vi "Abort All Top Level in App Instance.vi"() -> ()   [LabVIEW 2020]
panel:
  in  "Select":bool
  in  "Contexts":i32(listbox)
  out "error out":errorcluster
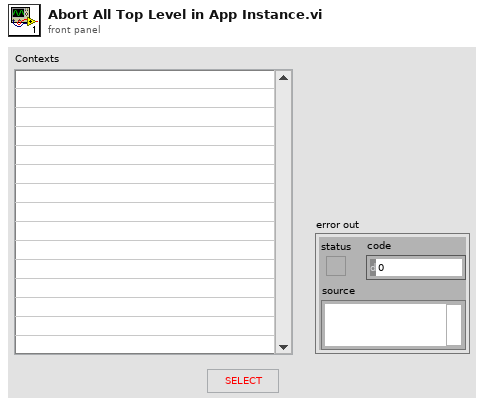
[diagram p1: front panel]
types:
  T1 = enum32{"Bad", "Idle", "Run top level", "Running"}
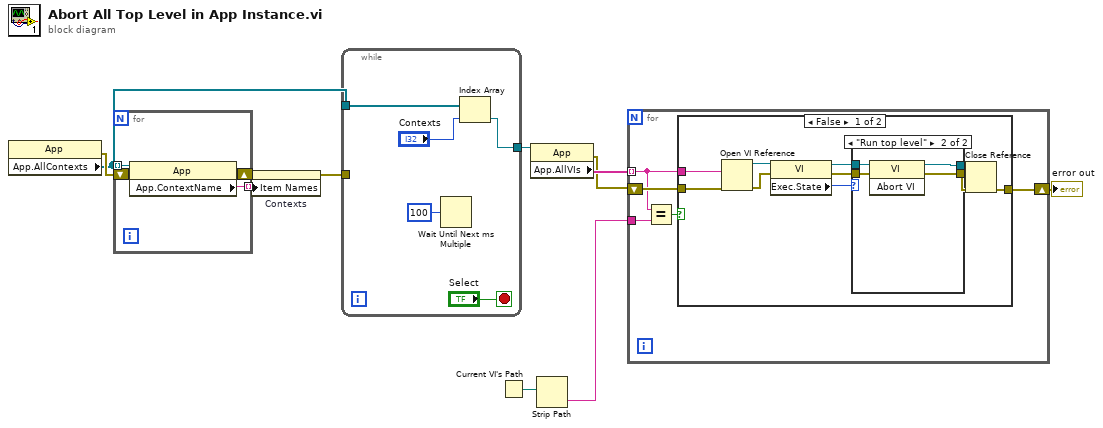
[diagram p0: block diagram]
diagram:
  n1 = property class="App"() -> (error out=w7:errorcluster, "App.AllContexts"=w4:refnum<vi>[])  [unwired: 2 in, 1 out]
  n2 = for {
    tunnel: w4 -> [w15] mode=indexing
    tunnel: [w14] -> w8 mode=indexing
    shift-right: [w12] -> w6
    shift-left: w7 -> [w13]
    n3 = property class="App"(reference=w15, error in=w13) -> (error out=w12:errorcluster, "App.ContextName"=w14:string)  [unwired: 1 out]
  }
  n4 = property on="Contexts" class="LstBox (strict)"(error in=w6, "Item Names"=w8) -> (error out=w5:errorcluster)  [unwired: 1 in, 1 out]
  n5 = while {
    tunnel: w5 -> [_]
    tunnel: w4 -> [w19]
    tunnel: [w17] -> w3
    stop <- "Select" stop-if-true
    n6 = Wait Until Next ms Multiple(millisecond multiple=u32 100) -> ()  [unwired: 1 out]
    n7 = Index Array(array=w19, index="Contexts") -> (element=w17:refnum<vi>)
  }
  n8 = Current VI's Path() -> (path=w2:path)
  n9 = property class="App"(reference=w3) -> (error out=w10:errorcluster, "App.AllVIs"=w11:string[])  [unwired: 1 in, 1 out]
  n10 = Strip Path(path=w2) -> (name=w1:string)  [unwired: 1 out]
  n11 = for {
    tunnel: w11 -> [w22] mode=indexing
    shift-right: [w24] -> w9
    shift-left: w10 -> [w25]
    tunnel: w1 -> [w23]
    n12 = Equal?(x=w22, y=w23) -> (x = y?=w21:bool)
    n13 = case shown="False" w21 {
      tunnel: w25 -> [w28 w42]
      tunnel: [w27 w42] -> w24
      tunnel: w22 -> [w26 _]
      frame False {
        n14 = Open VI Reference(vi path=w26, error in (no error)=w28) -> (vi reference=w35:refnum<vi>, error out=w34:errorcluster)  [unwired: 4 out]
        n15 = property class="VI"(reference=w35, error in=w34) -> (reference out=w31:refnum<vi>, error out=w32:errorcluster, "Exec.State"=w33:T1)
        n16 = case shown="\"Run top level\"" w33 {
          tunnel: w32 -> [w36 w41]
          tunnel: w31 -> [w37 w40]
          tunnel: [w37 w39] -> w29
          tunnel: [w36 w38] -> w30
          frame "Bad", Default {
          }
          frame "Run top level" {
            n17 = invoke class="VI" method="Abort VI"(reference=w40, error in=w41) -> (reference out=w39:refnum<vi>, error out=w38:errorcluster)  [unwired: 1 in, 1 out]
          }
        }
        n18 = Close Reference(reference=w29, error in (no error)=w30) -> (error out=w27:errorcluster)
      }
      frame True {
        # "Don't stop this VI."
      }
    }
  }
  "error out" <- w9
